vi "Generic GetTempTree - AI6.v.vi"(0 "MW100":refnum<visa-resource-name>, 2 "Semiphore":T1, 11 "Error In":errorcluster) -> (4 "dup VISA session":refnum<visa-resource-name>, 6 "Tc Tree":dbl[](array[numeric]) format="%.4f", 15 "error out":errorcluster)   [LabVIEW 2009]
uses:
  ChannelSettings.ctl
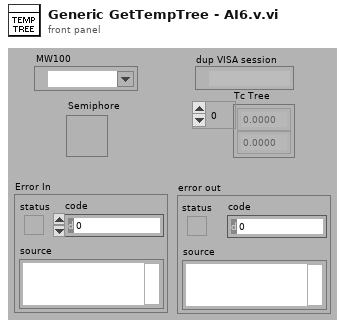
[diagram p1: front panel]
types:
  T1 = typedef "Semaphore RefNum" = refnum<k1>
  T2 = typedef "ChannelSettings.ctl" = u32
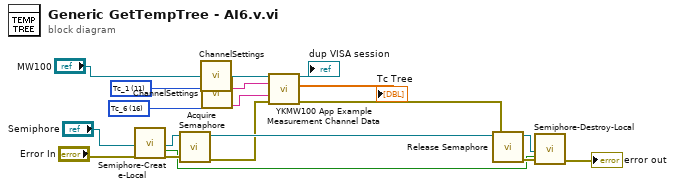
[diagram p0: block diagram]
diagram:
  w12 = T2 16 items=["4-20_OUT", "Pres_HI1", "Pres_HI2", "Pres_LOW", "Pres_PIN", "HEATER_TOP", "HEATER_BOT", "T_Shell", "FLOWMETER", "WATT_SENSE", "WH_TICK", "Tc_1", "Tc_2", "Tc_3", "Tc_4", "Tc_5", "Tc_6", "Tc_down", "T_Shell_2", "T_Shell_3", "T_Shell_4", "RTD_IN", "RTD_OUT", "RTD_AMB", "INTF_TEMPFLO", "INTF_READY", "INTF_START", "INTF_STOP", "DRM_LOW", "DRM_HIGH", "PWR_MAIN", "VLV_DUMP", "VLV_OUT", "VLV_IN", "WATT_HOURS", "FLOW(SAMPLE)", "GALLONS", "FLOW(GPM)"] ("Channel_Enum")
  w13 = T2 11 items=["4-20_OUT", "Pres_HI1", "Pres_HI2", "Pres_LOW", "Pres_PIN", "HEATER_TOP", "HEATER_BOT", "T_Shell", "FLOWMETER", "WATT_SENSE", "WH_TICK", "Tc_1", "Tc_2", "Tc_3", "Tc_4", "Tc_5", "Tc_6", "Tc_down", "T_Shell_2", "T_Shell_3", "T_Shell_4", "RTD_IN", "RTD_OUT", "RTD_AMB", "INTF_TEMPFLO", "INTF_READY", "INTF_START", "INTF_STOP", "DRM_LOW", "DRM_HIGH", "PWR_MAIN", "VLV_DUMP", "VLV_OUT", "VLV_IN", "WATT_HOURS", "FLOW(SAMPLE)", "GALLONS", "FLOW(GPM)"] ("Channel_Enum")
  n1 = call "Semiphore-Create-Local.vi"("Semiphore"="Semiphore", "error in (no error)"="Error In") -> ("semaphore"=w8:T1, "Local?"=w5:bool, "error out"=w10:errorcluster)  [unwired: 15 in]
  n2 = call <vilib>:"Acquire Semaphore.vi"("error in (no error)"=w10, "semaphore"=w8) -> ("error out"=w1:errorcluster, "semaphore out"=w11:T1)  [unwired: 3 in, 1 out]
  n3 = call "ChannelSettings.vi"("Channel_Enum"=w13) -> ("Channel String"=w18:string)  [unwired: 10 in]
  n4 = call "ChannelSettings.vi"("Channel_Enum"=w12) -> ("Channel String"=w14:string)  [unwired: 10 in]
  n5 = call <instrlib>:"YKMW100 App Example Measurement Channel Data.vi"("VISA session"="MW100", "Start Channel (001)"=w18, "End Channel (001)"=w14, "error in (no error)"=w1) -> ("dup VISA session"=→"dup VISA session":refnum<visa-resource-name>, "Data List"=→"Tc Tree":dbl[], "error out"=w2:errorcluster)  [unwired: 4 in, 5 out]
  n6 = call <vilib>:"Release Semaphore.vi"("error in (no error)"=w2, "semaphore"=w11) -> ("error out"=w7:errorcluster, "semaphore out"=w6:T1)  [unwired: 4 in]
  n7 = call "Semiphore-Destroy-Local.vi"("Semiphore"=w6, "Local?"=w5, "error in (no error)"=w7) -> ("error out"=→"error out":errorcluster)  [unwired: 16 in]
